vi "Initialize Attributes Core.vi"(8 "error in (no error)":errorcluster, 10 "Attribute Data":variant, 11 "BNT_DAQmx-MCSV in":refnum<class "BNT_DAQmx-MCSV.lvclass">) -> (0 "error out":errorcluster, 2 "MandatoryParameters":cluster{"Parameter":string, "found?":bool}[](array[cluster]), 3 "BNT_DAQmx-MCSV out":refnum<class "BNT_DAQmx-MCSV.lvclass">)   [LabVIEW 2018, in "BNT_DAQmx.lvlib" / "BNT_DAQmx-MCSV.lvclass"]
doc: "Initialize object attribute.\n\nUnique resources should be allocated elsewhere!"
uses:
  BNT_DAQmx-MCSV.lvclass
  C:/Users/Holger/Documents/LVP/HEITRONICS/TempCtrl/Packages/CSPP_Core/Actors/CSPP_DeviceActor/CSPP_DeviceActor.lvclass
  C:/Users/Holger/Documents/LVP/HEITRONICS/TempCtrl/Packages/CSPP_Core/Actors/CSPP_BaseActor/CSPP_BaseActor.lvclass
  CSPP_Core/Actors/CSPP_DeviceActor/CSPP_DeviceActor.lvclass/CSPP_DeviceActor.ctl
  CSPP_Core/Actors/CSPP_BaseActor/CSPP_BaseActor.lvclass/CSPP_BaseActor.ctl
  BNT_DAQmx-MCSV.lvclass/BNT_DAQmx-MCSV.ctl
  CSPP_Core/Actors/CSPP_DeviceActor/CSPP_DeviceActor.lvclass
  CSPP_Core/Classes/CSPP_BaseClasses/Factory/CSPP_Factory.lvclass
  CSPP_Core/Actors/CSPP_BaseActor/CSPP_BaseActor.lvclass
  CSPP_Core/Libraries/Utilities/CSPP_Utilities.lvlib
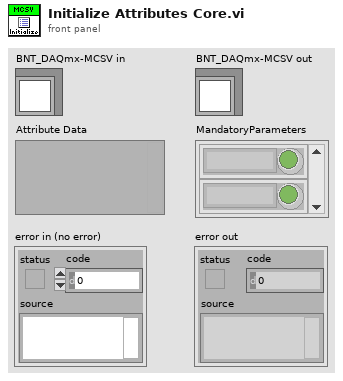
[diagram p1: front panel]
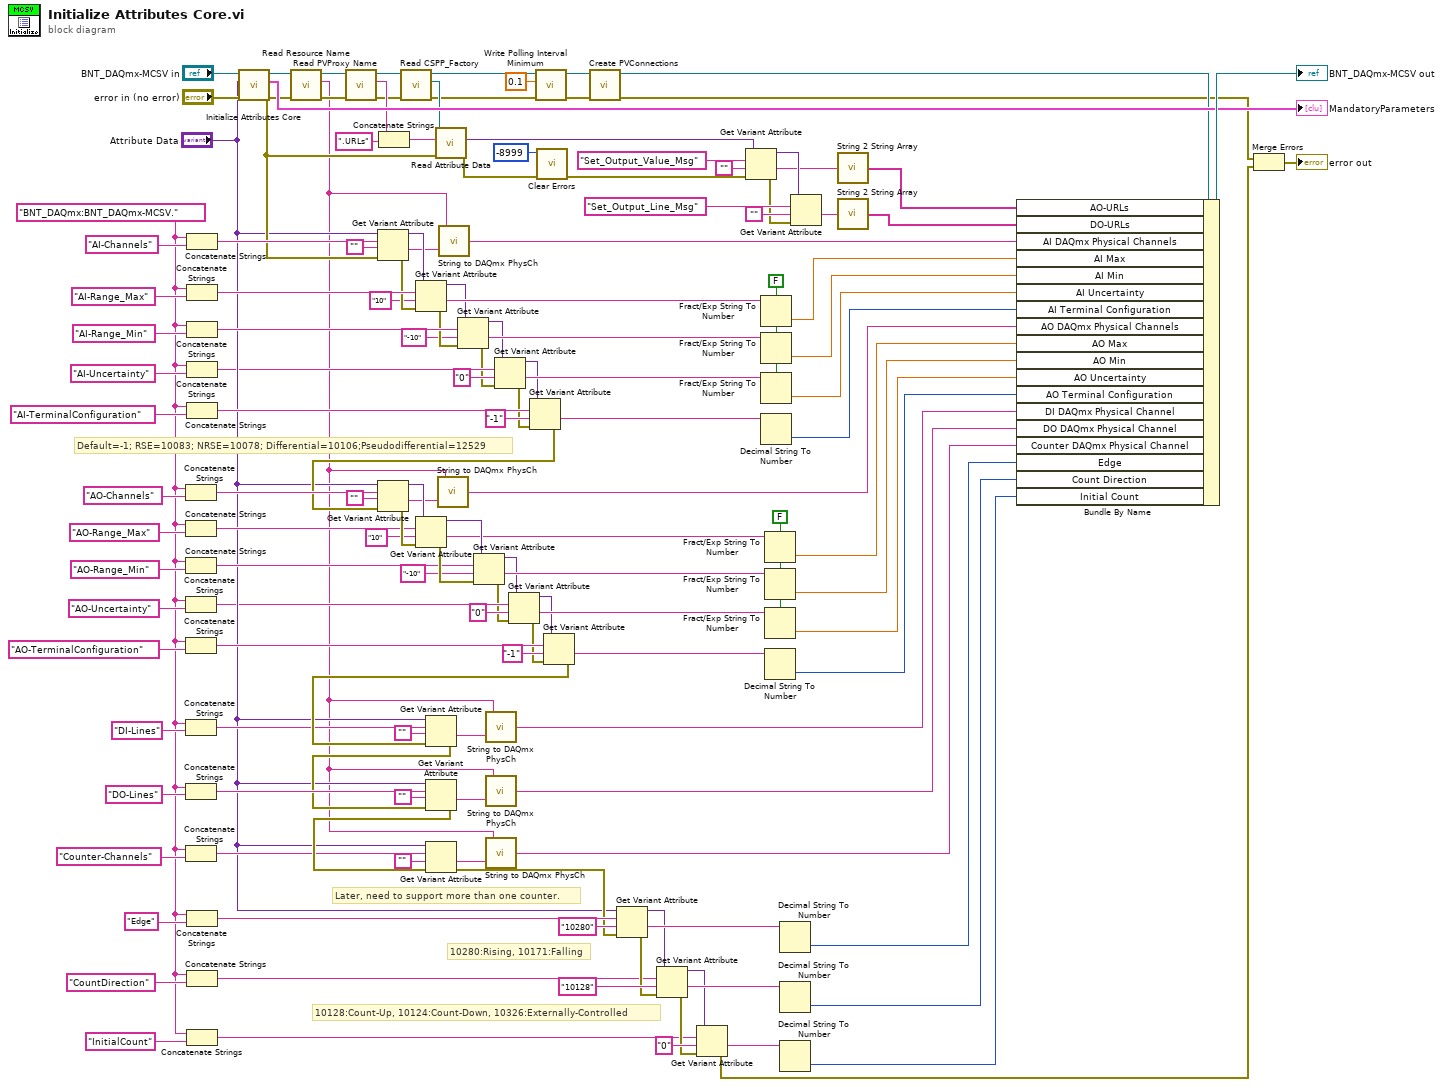
[diagram p0: block diagram]
diagram:
  w10 = FALSE ("use system decimal point (T)")
  w20 = FALSE ("use system decimal point (T)")
  w6 = "BNT_DAQmx:BNT_DAQmx-MCSV."
  # "Later, need to support more than one counter."
  # "10128:Count-Up, 10124:Count-Down, 10326:Externally-Controlled"
  # "10280:Rising, 10171:Falling"
  # "Default=-1; RSE=10083; NRSE=10078; Differential=10106;Pseudodifferential=12529"
  n1 = Concatenate Strings(w6, "AO-Channels" ("string")) -> (w122:string)
  n2 = Concatenate Strings(w6, "AO-Range_Max" ("string")) -> (w113:string)
  n3 = Concatenate Strings(w6, "AO-Range_Min" ("string")) -> (w116:string)
  n4 = Concatenate Strings(w6, "AO-Uncertainty" ("string")) -> (w12:string)
  n5 = Concatenate Strings(w6, "AO-TerminalConfiguration" ("string")) -> (w119:string)
  n6 = Concatenate Strings(w6, "DI-Lines" ("string")) -> (w100:string)
  n7 = Concatenate Strings(w6, "DO-Lines" ("string")) -> (w101:string)
  n8 = Concatenate Strings(w6, "Counter-Channels" ("string")) -> (w51:string)
  n9 = Concatenate Strings(w6, "AI-Channels" ("string")) -> (w130:string)
  n10 = Concatenate Strings(w6, "AI-Range_Max" ("string")) -> (w142:string)
  n11 = Concatenate Strings(w6, "AI-Range_Min" ("string")) -> (w139:string)
  n12 = Concatenate Strings(w6, "AI-Uncertainty" ("string")) -> (w22:string)
  n13 = Concatenate Strings(w6, "AI-TerminalConfiguration" ("string")) -> (w136:string)
  n14 = Concatenate Strings(w6, "Edge" ("string")) -> (w63:string)
  n15 = Concatenate Strings(w6, "CountDirection" ("string")) -> (w58:string)
  n16 = Concatenate Strings(w6, "InitialCount" ("string")) -> (w60:string)
  n17 = call-parent "Initialize Attributes Core.vi"("error in (no error)"="error in (no error)", "Attribute Data"="Attribute Data", "CSPP_DeviceActor in"="BNT_DAQmx-MCSV in") -> ("error out"=w42:errorcluster, "MandatoryParameters"=→"MandatoryParameters":cluster{"Parameter":string, "found?":bool}[], "CSPP_DeviceActor out"=w126:refnum<class "BNT_DAQmx-MCSV.lvclass">)  [unwired: 6 in]
  n18 = call "Read Resource Name.vi"("error in (no error)"=w42, "CSPP_DeviceActor in"=w126) -> ("error out"=w43:errorcluster, "Resource Name"=w2:string, "CSPP_DeviceActor out"=w98:refnum<class "BNT_DAQmx-MCSV.lvclass">)  [unwired: 7 in]
  n19 = call "Read PVProxy Name.vi"("error in (no error)"=w43, "CSPP_BaseActor in"=w98) -> ("error out"=w35:errorcluster, "PVProxy Name"=w93:string, "CSPP_BaseActor out"=w38:refnum<class "BNT_DAQmx-MCSV.lvclass">)  [unwired: 7 in]
  n20 = Get Variant Attribute(Variant="Attribute Data", name=w130, default value (empty Variant)="", error in=w42) -> (duplicate Variant=w129:variant, value=w1:string, error out=w128:errorcluster)  [unwired: 1 out]
  n21 = Concatenate Strings(w93, ".URLs" ("string")) -> (w95:string)
  n22 = call "Read CSPP_Factory.vi"("error in (no error)"=w35, "CSPP_BaseActor in"=w38) -> ("error out"=w34:errorcluster, "CSPP_Factory"=w36:refnum<class "CSPP_Factory.lvclass">, "CSPP_BaseActor out"=w37:refnum<class "BNT_DAQmx-MCSV.lvclass">)  [unwired: 7 in]
  n23 = Get Variant Attribute(Variant=w129, name=w142, default value (empty Variant)="10" ("string"), error in=w128) -> (duplicate Variant=w140:variant, value=w141:string, error out=w138:errorcluster)  [unwired: 1 out]
  n24 = call-dynamic "Read Attribute Data.vi"("error in (no error)"=w42, "Object Name"=w95, "CSPP_Factory in"=w36) -> ("error out"=w97:errorcluster, "Attribute Data"=w91:variant)  [unwired: 6 in, 1 out]
  n25 = call "String to DAQmx PhysCh.vi"("Channel String"=w1, "Resource Name"=w2) -> ("DAQmx Physical Channels"=w3:string)
  n26 = Get Variant Attribute(Variant=w140, name=w139, default value (empty Variant)="-10" ("string"), error in=w138) -> (duplicate Variant=w17:variant, value=w137:string, error out=w16:errorcluster)  [unwired: 1 out]
  n27 = Get Variant Attribute(Variant=w17, name=w22, default value (empty Variant)="0" ("string"), error in=w16) -> (duplicate Variant=w19:variant, value=w23:string, error out=w18:errorcluster)  [unwired: 1 out]
  n28 = Get Variant Attribute(Variant=w19, name=w136, default value (empty Variant)="-1" ("string"), error in=w18) -> (value=w135:string, error out=w108:errorcluster)  [unwired: 2 out]
  n29 = Get Variant Attribute(Variant="Attribute Data", name=w122, default value (empty Variant)="", error in=w108) -> (duplicate Variant=w123:variant, value=w32:string, error out=w124:errorcluster)  [unwired: 1 out]
  n30 = Get Variant Attribute(Variant=w123, name=w113, default value (empty Variant)="10" ("string"), error in=w124) -> (duplicate Variant=w115:variant, value=w114:string, error out=w117:errorcluster)  [unwired: 1 out]
  n31 = call "String to DAQmx PhysCh.vi"("Channel String"=w32, "Resource Name"=w2) -> ("DAQmx Physical Channels"=w31:string)
  n32 = Get Variant Attribute(Variant=w115, name=w116, default value (empty Variant)="-10" ("string"), error in=w117) -> (duplicate Variant=w5:variant, value=w118:string, error out=w4:errorcluster)  [unwired: 1 out]
  n33 = Get Variant Attribute(Variant=w5, name=w12, default value (empty Variant)="0" ("string"), error in=w4) -> (duplicate Variant=w8:variant, value=w11:string, error out=w7:errorcluster)  [unwired: 1 out]
  n34 = call "Write Polling Interval Minimum.vi"("error in (no error)"=w34, "Polling Interval Minimum"=dbl[unit] 0.1, "CSPP_BaseActor in"=w37) -> ("error out"=w44:errorcluster, "CSPP_BaseActor out"=w46:refnum<class "BNT_DAQmx-MCSV.lvclass">)  [unwired: 7 in]
  n35 = call <vilib>:"Clear Errors.vi"("error in (no error)"=w97, "specific error code to clear (0: all)"=-8999) -> ("error out"=w90:errorcluster)  [unwired: 4 in, 1 out]
  n36 = Get Variant Attribute(Variant=w8, name=w119, default value (empty Variant)="-1" ("string"), error in=w7) -> (value=w120:string, error out=w105:errorcluster)  [unwired: 2 out]
  n37 = Get Variant Attribute(Variant="Attribute Data", name=w100, default value (empty Variant)="", error in=w105) -> (value=w30:string, error out=w99:errorcluster)  [unwired: 2 out]
  n38 = Get Variant Attribute(Variant="Attribute Data", name=w101, default value (empty Variant)="", error in=w99) -> (value=w28:string, error out=w53:errorcluster)  [unwired: 2 out]
  n39 = Get Variant Attribute(Variant="Attribute Data", name=w51, default value (empty Variant)="", error in=w53) -> (value=w26:string, error out=w54:errorcluster)  [unwired: 2 out]
  n40 = call "String to DAQmx PhysCh.vi"("Channel String"=w30, "Resource Name"=w2) -> ("DAQmx Physical Channels"=w29:string)
  n41 = call "String to DAQmx PhysCh.vi"("Channel String"=w28, "Resource Name"=w2) -> ("DAQmx Physical Channels"=w27:string)
  n42 = call "String to DAQmx PhysCh.vi"("Channel String"=w26, "Resource Name"=w2) -> ("DAQmx Physical Channels"=w25:string)
  n43 = call "Create PVConnections.vi"("error in (no error)"=w44, "BNT_DAQmx-MCSV in"=w46) -> ("error out"=w41:errorcluster, "BNT_DAQmx-MCSV out"=w45:refnum<class "BNT_DAQmx-MCSV.lvclass">)  [unwired: 8 in]
  n44 = Get Variant Attribute(Variant="Attribute Data", name=w63, default value (empty Variant)="10280", error in=w54) -> (duplicate Variant=w52:variant, value=w65:string, error out=w64:errorcluster)  [unwired: 1 out]
  n45 = Get Variant Attribute(Variant=w52, name=w58, default value (empty Variant)="10128", error in=w64) -> (duplicate Variant=w59:variant, value=w68:string, error out=w61:errorcluster)  [unwired: 1 out]
  n46 = Get Variant Attribute(Variant=w59, name=w60, default value (empty Variant)="0", error in=w61) -> (value=w69:string, error out=w40:errorcluster)  [unwired: 2 out]
  n47 = Get Variant Attribute(Variant=w91, name="Set_Output_Value_Msg", default value (empty Variant)="", error in=w90) -> (duplicate Variant=w86:variant, value=w84:string, error out=w85:errorcluster)  [unwired: 1 out]
  n48 = Fract/Exp String To Number(use system decimal point (T)=w20, string=w141) -> (number=w80:dbl)  [unwired: 2 in, 1 out]
  n49 = Fract/Exp String To Number(use system decimal point (T)=w20, string=w137) -> (number=w79:dbl)  [unwired: 2 in, 1 out]
  n50 = Fract/Exp String To Number(use system decimal point (T)=w20, string=w23) -> (number=w15:dbl)  [unwired: 2 in, 1 out]
  n51 = Decimal String To Number(string=w135) -> (number=w133:i32)  [unwired: 2 in, 1 out]
  n52 = Fract/Exp String To Number(use system decimal point (T)=w10, string=w114) -> (number=w78:dbl)  [unwired: 2 in, 1 out]
  n53 = Fract/Exp String To Number(use system decimal point (T)=w10, string=w118) -> (number=w77:dbl)  [unwired: 2 in, 1 out]
  n54 = Fract/Exp String To Number(use system decimal point (T)=w10, string=w11) -> (number=w9:dbl)  [unwired: 2 in, 1 out]
  n55 = Decimal String To Number(string=w120) -> (number=w109:i32)  [unwired: 2 in, 1 out]
  n56 = Decimal String To Number(string=w65) -> (number=w49:i32)  [unwired: 2 in, 1 out]
  n57 = Decimal String To Number(string=w68) -> (number=w48:i32)  [unwired: 2 in, 1 out]
  n58 = Decimal String To Number(string=w69) -> (number=w47:i32)  [unwired: 2 in, 1 out]
  n59 = Get Variant Attribute(Variant=w86, name="Set_Output_Line_Msg", default value (empty Variant)="", error in=w85) -> (value=w83:string)  [unwired: 3 out]
  n60 = call "String 2 String Array.vi"("String"=w84) -> ("Substrings"=w82:string[])  [unwired: 1 in]
  n61 = call "String 2 String Array.vi"("String"=w83) -> ("Substrings"=w81:string[])  [unwired: 1 in]
  n62 = Bundle By Name(cluster=w45, "AO-URLs"=w82, "DO-URLs"=w81, "AI DAQmx Physical Channels"=w3, "AI Max"=w80, "AI Min"=w79, "AI Uncertainty"=w15, "AI Terminal Configuration"=w133, "AO DAQmx Physical Channels"=w31, "AO Max"=w78, "AO Min"=w77, "AO Uncertainty"=w9, "AO Terminal Configuration"=w109, "DI DAQmx Physical Channel"=w29, "DO DAQmx Physical Channel"=w27, "Counter DAQmx Physical Channel"=w25, "Edge"=w49, "Count Direction"=w48, "Initial Count"=w47) -> (→"BNT_DAQmx-MCSV out":refnum<class "BNT_DAQmx-MCSV.lvclass">)
  n63 = Merge Errors(w41, w40) -> (→"error out":errorcluster)
